vi "UTEX Read VISA.vi"(8 "error in":errorcluster, 10 "write buffer":string, 11 "VISA Refnum in":refnum<visa-resource-name>) -> (0 "error out":errorcluster, 2 "read buffer":string, 3 "VISA Refnum out":refnum<visa-resource-name>)   [LabVIEW 2022 SP3]
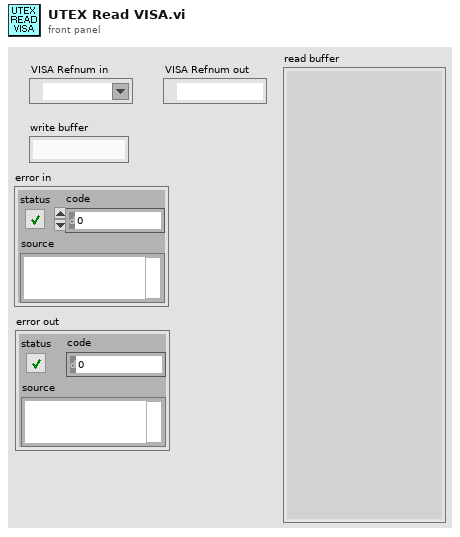
[diagram p1: front panel]
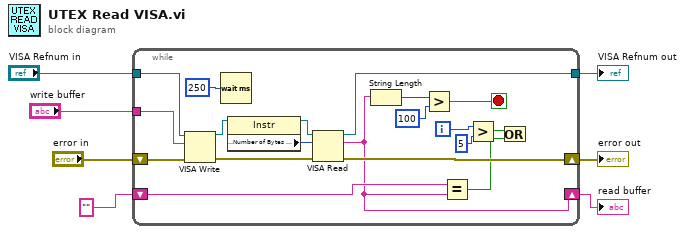
[diagram p0: block diagram]
diagram:
  n1 = while {
    tunnel: "write buffer" -> [w23]
    tunnel: "VISA Refnum in" -> [w22]
    shift-right: [w26] -> w2
    shift-left: "error in" -> [w24]
    shift-right: [w12] -> w6
    shift-left: "" ("read buffer") -> [w16]
    tunnel: [w13] -> w7
    i -> [w15]
    stop <- w8 stop-if-true
    n2 = VISA Write(VISA resource name=w22, write buffer=w23, error in (no error)=w24) -> (VISA resource name out=w21:refnum<visa-resource-name>, error out=w25:errorcluster)  [unwired: 1 out]
    n3 = Wait (ms)(milliseconds to wait=u32 250) -> ()  [unwired: 1 out]
    n4 = property class="Instr"(reference=w21) -> (reference out=w19:refnum<visa-resource-name>, "Serial Settings:Number of Bytes at Serial Port"=w20:u32)  [unwired: 1 in, 1 out]
    n5 = VISA Read(VISA resource name=w19, byte count=w20, error in (no error)=w25) -> (VISA resource name out=w13:refnum<visa-resource-name>, read buffer=w12:string, error out=w26:errorcluster)  [unwired: 1 out]
    n6 = String Length(string=w12) -> (length=w11:i32)
    n7 = Greater?(x=w11, y=100 ("x")) -> (0:w8:bool)
    n8 = Equal?(x=w16, y=w12) -> (x = y?=w17:bool)
    n9 = Greater?(x=w15, y=5) -> (0:w9:bool)
    n10 = Or(x=w9, y=w17) -> ()  [unwired: 1 out]
  }
  "VISA Refnum out" <- w7
  "read buffer" <- w6
  "error out" <- w2
